vi "Synchronize X axis.vi"(4 "error in":errorcluster, 5 "input cluster":T1, 7 "Start (T) / Stop (F)":bool) -> (0 "error out":errorcluster, 1 "output cluster":T1)   [LabVIEW 2010]
uses:
  Main_cluster.ctl
  <vilib>/vision/Image Controls.llb/IMAQ Image.ctl
  <vilib>/DAQmx/configure/timing.llb/DAQmx Timing (Sample Clock).vi
  <vilib>/DAQmx/configure/timing.llb/DAQmx Timing (Implicit).vi
  C:/Program Files (x86)/National Instruments/LabVIEW 2010/resource/objmgr/daqmx.rc
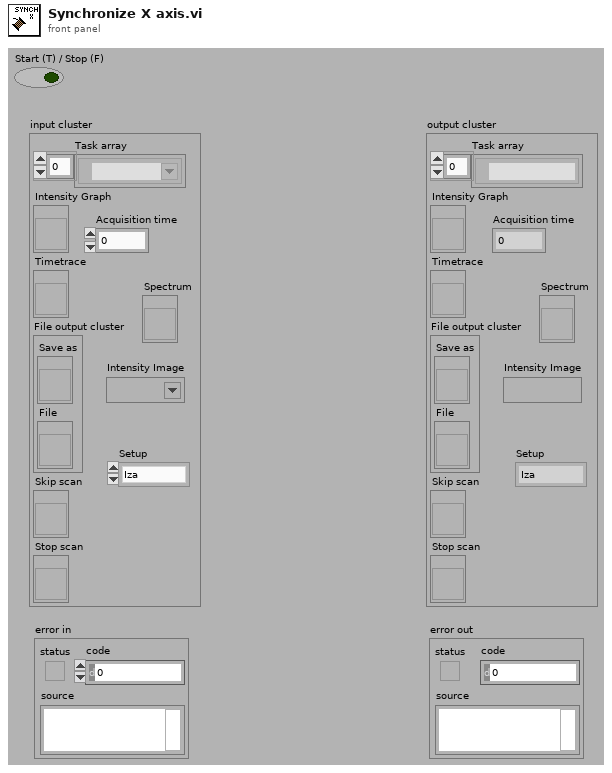
[diagram p1: front panel]
types:
  T1 = typedef "Main_cluster.ctl" = cluster{"Task array":refnum<k21>[], "Intensity Graph":refnum<vi>, "Timetrace":refnum<vi>, "File output cluster":cluster{"Save as":refnum<vi>, "File":refnum<vi>}, "Skip scan":refnum<vi>, "Stop scan":refnum<vi>, "Acquisition time":dbl, "Setup":enum16{"Iza", "Lukasz"}, "Spectrum":refnum<vi>, "Intensity Image":T2}
  T2 = typedef "IMAQ Image.ctl" = refnum<image>
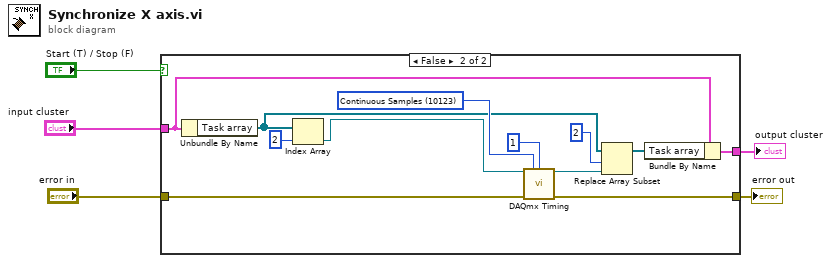
[diagram p0: block diagram]
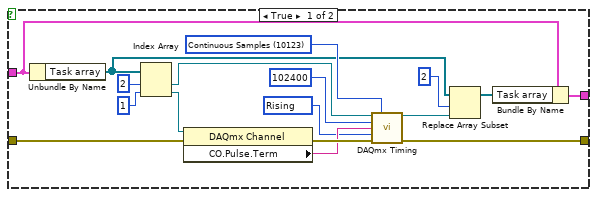
[diagram p2: hidden frame]
diagram:
  n1 = case shown="False" "Start (T) / Stop (F)" {
    tunnel: [w22 w34] -> w5
    tunnel: [w21 w33] -> w4
    tunnel: "input cluster" -> [w20 w32]
    tunnel: "error in" -> [w19 w24]
    frame True {
      w11 = 10123 items=["Finite Samples"=10178, "Continuous Samples"=10123, "Hardware Timed Single Point"=12522] ("sample mode")
      w12 = 10280 items=["Rising"=10280, "Falling"=10171] ("active edge")
      n2 = Unbundle By Name(w20) -> ("Task array"=w10:refnum<k21>[])
      n3 = Index Array(array=w10, index #1=2 ("index"), index #2=1 ("index")) -> (element #1=w17:refnum<k21>, element #2=w15:refnum<k21>)
      n4 = property class="DAQmx Channel"(reference=w15, error in=w19) -> (error out=w14:errorcluster, "CO.Pulse.Term"=w13:tag)  [unwired: 1 out]
      n5 = call-poly <vilib>:"DAQmx Timing.vi"("task/channels in"=w17, "sample mode"=w11, "rate"=102400 ("samples per channel"), "source"=w13, "active edge"=w12, "error in"=w14) -> ("task out"=w8:refnum<k21>, "error out"=w22:errorcluster)  [unwired: 8 in]
      n6 = Replace Array Subset(array=w10, new element=w8, index=2) -> (w7:refnum<k21>[])
      n7 = Bundle By Name(cluster=w20, "Task array"=w7) -> (w21:T1)
    }
    frame False {
      w29 = 10123 items=["Finite Samples"=10178, "Continuous Samples"=10123, "Hardware Timed Single Point"=12522] ("sample mode")
      n8 = Unbundle By Name(w32) -> ("Task array"=w28:refnum<k21>[])
      n9 = Index Array(array=w28, index=2) -> (element=w30:refnum<k21>)
      n10 = call-poly <vilib>:"DAQmx Timing.vi"("task/channels in"=w30, "sample mode"=w29, "samples per channel"=1, "error in"=w24) -> ("task out"=w26:refnum<k21>, "error out"=w34:errorcluster)  [unwired: 10 in]
      n11 = Replace Array Subset(array=w28, new element=w26, index=2) -> (w25:refnum<k21>[])
      n12 = Bundle By Name(cluster=w32, "Task array"=w25) -> (w33:T1)
    }
  }
  "error out" <- w5
  "output cluster" <- w4
